vi "subvi_List Folders.vi"(7 "root path":path, 8 "error in (no error)":errorcluster, 9 "folder names":string[](array[string]), 11 "path":path) -> (0 "error out":errorcluster, 2 "Path Strings":string[](array[string]), 3 "Paths":path[](array[path]))   [LabVIEW 2015, in "File Version Lib.lvlib"]
uses:
  File Version Lib.lvlib
  <userlib>/_OpenG.lib/file/file.llb/Compare Two Paths - Scalar__ogtk.vi
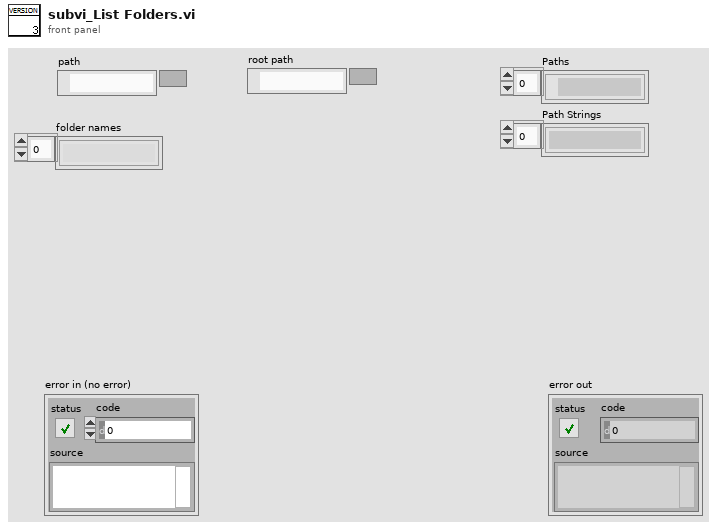
[diagram p1: front panel]
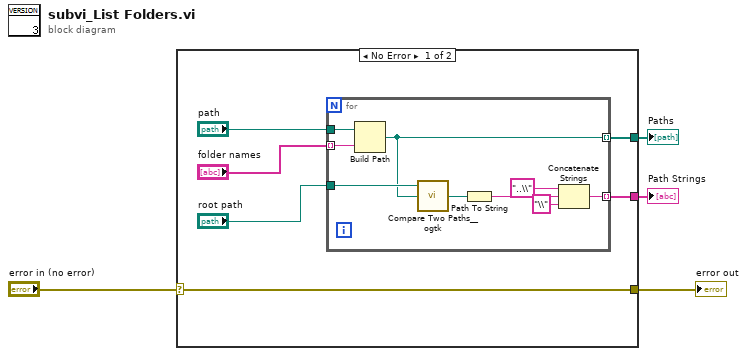
[diagram p0: block diagram]
diagram:
  n1 = case shown="No Error" "error in (no error)" {
    selector: "error in (no error)" -> [w10 w20]
    tunnel: [w10 w20] -> w3
    tunnel: [w6 _] -> w2
    tunnel: [w5 _] -> w1
    frame No Error {
      n2 = for {
        tunnel: "path" -> [w19]
        tunnel: "folder names" -> [w18] mode=indexing
        tunnel: [w16] -> w6 mode=indexing
        tunnel: "root path" -> [w17]
        tunnel: [w13] -> w5 mode=indexing
        n3 = Build Path(base path=w19, name or relative path=w18) -> (appended path=w16:path)
        n4 = call-poly <userlib>:"Compare Two Paths__ogtk.vi"("path2"=w16, "path1"=w17) -> ("relative path from 1 to 2"=w15:path)  [unwired: 1 in, 2 out]
        n5 = Path To String(path=w15) -> (string=w14:string)
        n6 = Concatenate Strings("..\\" ("string"), w14, "\\" ("string")) -> (w13:string)
      }
    }
    frame Error {
    }
  }
  "error out" <- w3
  "Paths" <- w2
  "Path Strings" <- w1
